vi "FPGA_Readout.vi"() -> ()   [LabVIEW 2020]
uses:
  <vilib>/Platform/TimedLoop/XDataNode/timing_clust.ctl
  <vilib>/Platform/TimedLoop/XDataNode/nitl_modes.ctl
  <vilib>/Platform/TimedLoop/XDataNode/wakeup.ctl
  <vilib>/rvi/Emulation/niFpgaGetClockAttributes.vi
  <vilib>/rvi/Emulation/niFpgaSctlEmulationGetInTimedLoop.vi
  <vilib>/rvi/Emulation/niFpgaEmulationReportErrorSimple.vi
  <vilib>/rvi/Emulation/niFpgaCriticalErrorInLSC.vi
  <vilib>/rvi/eio/common/nirviEmuTemplateMethod_errors.vi
  <vilib>/rvi/Emulation/niFpgaProcessEmulError.vi
  <vilib>/rvi/interface/RandomDataEmulation/niFpgaRandomDataHandleErrors.vi
  <vilib>/Platform/TimedLoop/XDataNode/XDataNode.xnode
  <vilib>/eio/EIONode/EIONode.xnode
  <vilib>/rvi/DataTransferAndStorage/Container/XNode/niFpgaContainer.xnode
  <vilib>/rvi/interface/RandomDataEmulation/nirviRandomDataFpgaReadWriteTemplate.vi
  <vilib>/Platform/TimedLoop/XDataNode/XDNodeRunTimeDep.lvlib
panel:
  out "Numeric":i32
  out "TargetToHostTimeout":bool
  out "Photon Count":u32
  in  "Reset Counter":bool
  in  "stop":bool
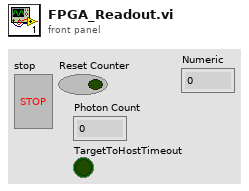
[diagram p1: front panel]
types:
  T1 = typedef "XDNodeRunTimeDep.lvlib/timing_clust.ctl" = cluster{"Expected End [f-1]":u64, "Actual End [f-1]":u64, "Finished Late? [f-1]":bool, "Expected End [i-1]":u64, "Actual End [i-1]":u64, "Finished Late? [i-1]":bool, "Expected Start [i]":u64, "Actual Start [i]":u64, "Expected Start [f]":u64, "Actual Start [f]":u64, "Source Name":string, "Structure Name":string, "Period":i64, "Deadline":i64, "Offset":i64, "Start":i64, "Priority":i32, "Timeout":i32, "Mode":T2, "Wakeup Reason":T3, "Error":errorcluster, "Source Type":string, "Secondary Source Type":string, "Global End Time":u64, "Global Start Time":u64, "Frame Duration":u64, "Iteration Duration":u64, "Assigned CPU":i32, "I/O Scan Engine Mode":u32}
  T2 = typedef "XDNodeRunTimeDep.lvlib/nitl_modes.ctl" = enum32{"No Change", "Process missed periods, maintain original phase", "Discard missed periods, maintain original phase", "Process missed periods, ignore original phase", "Discard missed periods, ignore original phase"}
  T3 = typedef "XDNodeRunTimeDep.lvlib/wakeup.ctl" = enum32{"Normal", "Aborted", "Asynchronous wakeup", "Timing source error", "Timed loop error", "Timeout"}
  T4 = enum16{"Rising Edge", "Falling Edge", "Rising AND Falling Edges"}
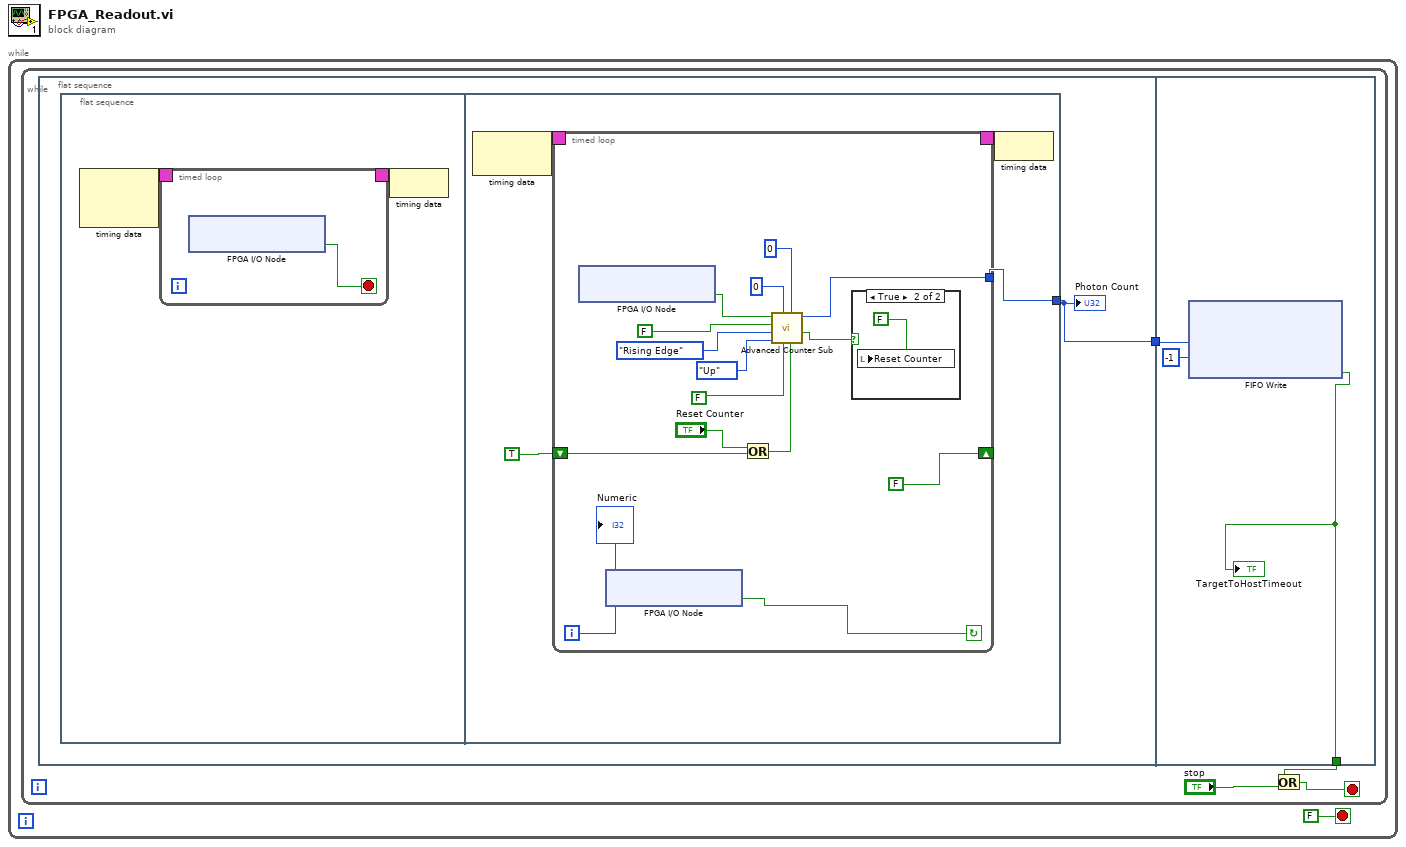
[diagram p0: block diagram]
diagram:
  n1 = while {
    stop <- FALSE stop-if-true
    n2 = while {
      stop <- w4 stop-if-true
      n3 = flat-sequence {
        tunnel: [w6] -> w3
        tunnel: w3 -> [w40]
        tunnel: [w38] -> w2
        frame #0 {
          n4 = flat-sequence {
            tunnel: [w14] -> w6
            frame #0 {
              n5 = node-c288() -> (w8:T1)  [unwired: 2 in]
              n6 = timed-loop {
                timing: w8 -> [_]
                timing-out: [_] -> w7
                stop <- w9 stop-if-true
                n7 = xnode "FPGA I/O Node"() -> ("Connector0/DIO4"=w9:bool)  [unwired: 1 in, 1 out]
              }
              n8 = node-c288(w7) -> ()
            }
            frame #1 {
              n9 = node-c288() -> (w17:T1)  [unwired: 1 in]
              n10 = timed-loop {
                timing: w17 -> [_]
                timing-out: [_] -> w16
                tunnel: [w21] -> w14
                shift-right: [FALSE] -> _
                shift-left: TRUE -> [w32]
                i -> [w19]
                stop <- w18 continue-if-true
                n11 = xnode "FPGA I/O Node"() -> ("Connector0/DIO0"=w25:bool)  [unwired: 1 in, 1 out]
                n12 = xnode "FPGA I/O Node"() -> ("Connector0/DIO4"=w18:bool)  [unwired: 1 in, 1 out]
                n13 = Or(x="Reset Counter", y=w32) -> (x .or. y?=w30:bool)
                n14 = call "Advanced Counter Sub.vi"("Reset Counter"=w30, "Init Counter Value"=u32 0, "Enable HW Gate"=FALSE, "Ticks to Filter"=u32 0, "Count Direction"=enum16{"Up", "Down"}."Up", "Edge"=T4."Rising Edge", "Gate Signal"=FALSE, "Input Signal"=w25) -> ("Counter Reset?"=w22:bool, "Counter Out"=w21:u32)  [unwired: 2 in]
                n15 = case shown="True" w22 {
                  frame False {
                  }
                  frame True {
                    n16 = local write "Reset Counter"(FALSE) -> ()
                  }
                }
                "Numeric" <- w19
              }
              n17 = node-c288(w16) -> ()
            }
          }
          "Photon Count" <- w6
        }
        frame #1 {
          n18 = xnode ("FIFO Write")("Element"=w40, "Timeout"=-1) -> ("Timed Out?"=w38:bool)  [unwired: 1 in, 1 out]
          "TargetToHostTimeout" <- w38
        }
      }
      n19 = Or(x=w2, y="stop") -> (x .or. y?=w4:bool)
    }
  }
